vi "Connection Open.vi"(8 "error in (no error)":errorcluster, 11 "Conection Data":T1={"VISA resource name"="COM4"}) -> (0 "error out":errorcluster, 3 "Conection Data Out":T1={"VISA resource name"="COM4"})   [LabVIEW 2014, in "SJ-210 Lib.lvlib"]
doc: "Abre el puerto COM que indica el usuario y setea valores por defecto al puerto."
uses:
  SJ-210 Lib.lvlib
  Typedef/Connection Data.ctl
  <vilib>/Instr/_visa.llb/VISA Configure Serial Port (Instr).vi
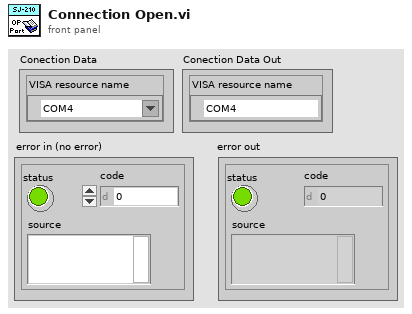
[diagram p1: front panel]
types:
  T1 = typedef "SJ-210 Lib.lvlib/Connection Data.ctl" = cluster{"VISA resource name":refnum<visa-resource-name>}
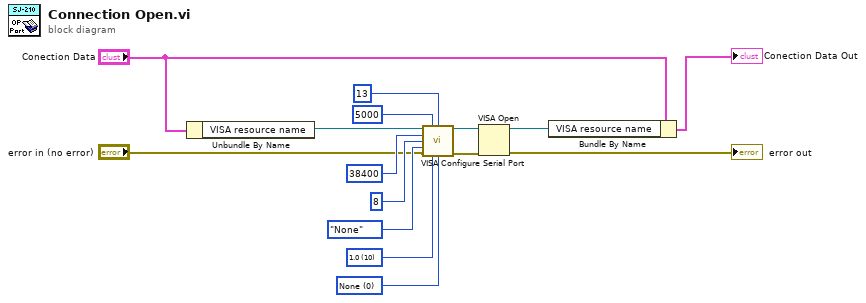
[diagram p0: block diagram]
diagram:
  w6 = u16 0 items=["None", "XON/XOFF", "RTS/CTS", "XON/XOFF & RTS/CTS", "DTR/DSR", "XON/XOFF & DTR/DSR"] ("flow control (0:none)")
  w7 = u16 10 items=["1.0"=10, "1.5"=15, "2.0"=20] ("stop bits (10: 1 bit)")
  n1 = Unbundle By Name("Conection Data") -> ("VISA resource name"=w3:refnum<visa-resource-name>)
  n2 = call-poly "VISA Configure Serial Port"("VISA resource name"=w3, "timeout (10sec)"=u32 5000, "termination char\n(0xA = '\\n' = LF)"=u8 13 ("termination char\n(0xA = '\\n' = LF)"), "baud rate (9600)"=u32 38400, "data bits (8)"=u16 8, "parity (0:none)"=enum16{"None", "Odd", "Even", "Mark", "Space"}."None", "error in (no error)"="error in (no error)", "stop bits (10: 1 bit)"=w7, "flow control (0:none)"=w6) -> ("VISA resource name out"=w5:refnum<visa-resource-name>, "error out"=w4:errorcluster)  [unwired: 5 in]
  n3 = VISA Open(error in (no error)=w4, VISA resource name=w5) -> (VISA resource name=w14:refnum<visa-resource-name>, error out=→"error out":errorcluster)  [unwired: 3 in]
  n4 = Bundle By Name(cluster="Conection Data", "VISA resource name"=w14) -> (→"Conection Data Out":T1)
